vi "atvaltas (SubVI).vi"(11 "m/s":dbl) -> (3 "km/h":dbl)   [LabVIEW 2015]
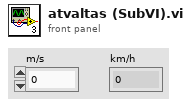
[diagram p1: front panel]
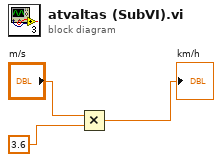
[diagram p0: block diagram]
diagram:
  n1 = Multiply(x="m/s", y=3.6) -> (x*y=→"km/h":dbl)
